vi "PH_ImageOperator.Draw Image.vi"(0 "i ref in":refnum<vi>, 2 "Cam Image":T1, 5 "error in (no error)":errorcluster) -> (14 "i ref out":refnum<vi>, 19 "error out":errorcluster)   [LabVIEW 2014, in "PH_ImageOperator.lvlib"]
doc: "This VI draws the image to the GUI. Depending on the sequencer state, it writes the images also to the attributes or calculates the pixel sum."
uses:
  PH_ImageOperator.lvlib
  <vilib>/vision/Image Controls.llb/IMAQ Image.ctl
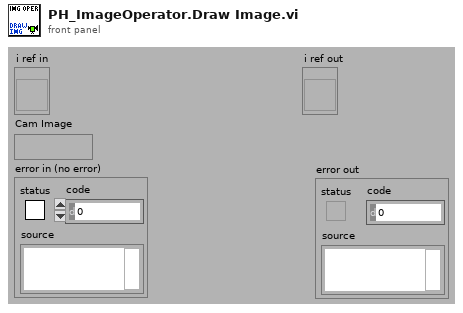
[diagram p1: front panel]
types:
  T1 = typedef "IMAQ Image.ctl" = refnum<image>
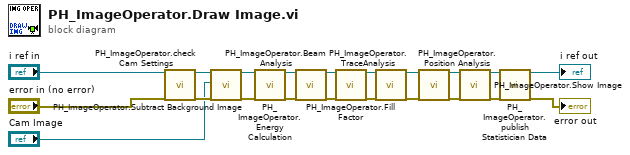
[diagram p0: block diagram]
diagram:
  n1 = call "PH_ImageOperator.check Cam Settings.vi"("i ref in"="i ref in", "error out"="error in (no error)") -> ("i ref out"=w16:refnum<vi>, "error out"=w15:errorcluster)  [unwired: 16 in]
  n2 = call "PH_ImageOperator.Subtract Background Image.vi"("i ref in"=w16, "Cam Image"="Cam Image", "error in (no error)"=w15) -> ("i ref out"=w14:refnum<vi>, "error out"=w13:errorcluster)  [unwired: 15 in]
  n3 = call "PH_ImageOperator.Energy Calculation.vi"("i ref in"=w14, "error in (no error)"=w13) -> ("i ref out"=w12:refnum<vi>, "error out"=w11:errorcluster)  [unwired: 16 in]
  n4 = call "PH_ImageOperator.Beam Analysis.vi"("i ref in"=w12, "error in (no error)"=w11) -> ("i ref out"=w6:refnum<vi>, "error out"=w4:errorcluster)  [unwired: 16 in]
  n5 = call "PH_ImageOperator.Fill Factor.vi"("i ref in"=w6, "error in"=w4) -> ("i ref out"=w5:refnum<vi>, "error out"=w3:errorcluster)  [unwired: 16 in]
  n6 = call "PH_ImageOperator.TraceAnalysis.vi"("i ref in"=w5, "error in (no error)"=w3) -> ("i ref out"=w8:refnum<vi>, "error out"=w10:errorcluster)  [unwired: 16 in]
  n7 = call "PH_ImageOperator.Position Analysis.vi"("i ref in"=w8, "error in (no error)"=w10) -> ("i ref out"=w7:refnum<vi>, "error out"=w9:errorcluster)  [unwired: 16 in]
  n8 = call "PH_ImageOperator.Show Image.vi"("i ref in"=w7, "error out"=w9) -> ("i ref out"=w2:refnum<vi>, "error out"=w17:errorcluster)  [unwired: 16 in]
  n9 = call "PH_ImageOperator.publish Statistician Data.vi"("i ref in"=w2, "error in"=w17) -> ("i ref out"=→"i ref out":refnum<vi>, "error out"=→"error out":errorcluster)  [unwired: 16 in]
